vi "Teleop.vi"(0 "Call Context":T9) -> (13 "SubState 3":T1, 14 "SubState 0":T5=enum."driver control", 15 "Loop 1 Data":T6, 16 "Loop 0 Data":T7, 17 "SubState 1":T5, 18 "Loop 2 Data":T4, 19 "SubState 2":T5)   [LabVIEW 2014]
uses:
  typedefs/state machine/subStates.ctl
  <vilib>/Rock Robotics/WPI/DriverStation/WPI_DriverStationDerivedRobotMode.ctl
  typedefs/loop datatypes/Loop 0 Datatype.ctl
  typedefs/drive mode.ctl
  typedefs/loop datatypes/Loop 1 Datatype.ctl
  typedefs/loop datatypes/Loop 2 Datatype.ctl
  <vilib>/Rock Robotics/WPI/Joystick/WPI_JoystickDevRef.ctl
  <vilib>/Rock Robotics/WPI/Joystick/WPI_JoystickDeviceEnum.ctl
  typedefs/state machine/singleUseSubstate.ctl
  typedefs/fg_getset.ctl
  typedefs/vision/vision enable.ctl
  global variables/devrefs.vi
panel:
  out "Drive to DC":bool
  out "JS3":T2={"Device"=enum."USB 1"}
  out "JS1":T2={"Device"=enum."USB 1"}
  out "JS2":T2={"Device"=enum."USB 1"}
  out "Exit Value":i32=-1
  # "Teleoperated Loop Data and Substates"
  # "Drive Loop"
  # "Loop 1: Lift"
  # "Loop 2: Container Arm"
  # "Loop 3: Tote Pistons"
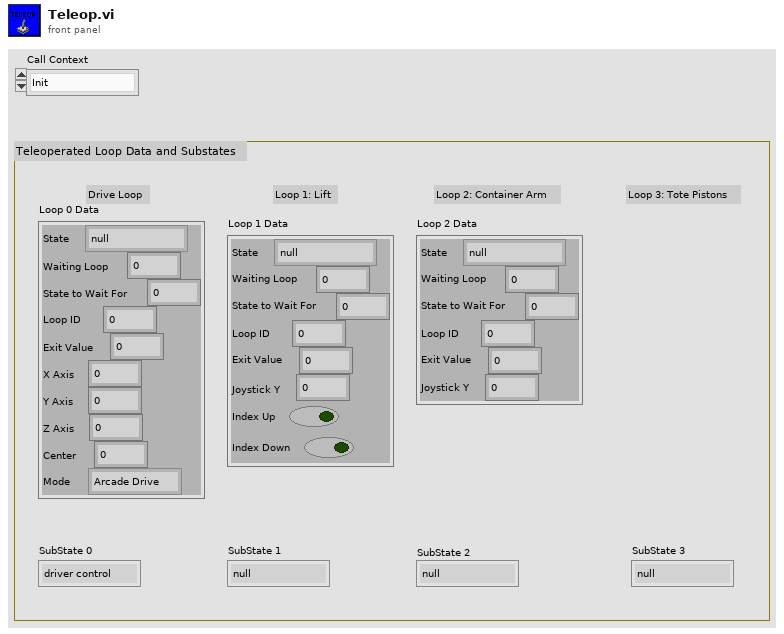
[diagram p1: front panel]
types:
  T1 = typedef "singleUseSubstate.ctl" = enum16{"null", "wait", "extend", "retract", "end"}
  T2 = typedef "WPI_JoystickDevRef.ctl" = cluster{"Device":T3}
  T3 = typedef "WPI_JoystickDeviceEnum.ctl" = enum16{"USB 0", "USB 1", "USB 2", "USB 3", "USB 4", "USB 5"}
  T4 = typedef "Loop 2 Datatype.ctl" = cluster{"State":T5, "Waiting Loop":i32, "State to Wait For":i32, "Loop ID":i32, "Exit Value":i32, "Joystick Y":dbl}
  T5 = typedef "subStates.ctl" = enum16{"null", "wait", "driver control", "auto", "manual override", "hold position", "rotate", "test", "end"}
  T6 = typedef "Loop 1 Datatype.ctl" = cluster{"State":T5, "Waiting Loop":i32, "State to Wait For":i32, "Loop ID":i32, "Exit Value":i32, "Joystick Y":dbl, "Index Up":bool, "Index Down":bool}
  T7 = typedef "Loop 0 Datatype.ctl" = cluster{"State":T5, "Waiting Loop":i32, "State to Wait For":i32, "Loop ID":i32, "Exit Value":i32, "X Axis":dbl, "Y Axis":dbl, "Z Axis":dbl, "Center":dbl, "Mode":T8}
  T8 = typedef "drive mode.ctl" = enum16{"Arcade Drive", "H-Drive", "H-Drive PID"}
  T9 = typedef "WPI_DriverStationDerivedRobotMode.ctl" = enum16{"Init", "Execute", "Stop"}
  T10 = cluster{"axis 1 (x)":dbl, "axis 2 (y)":dbl, "axis 3 (twist)":dbl, "axis 4 (throttle)":dbl, "axis 5":dbl, "axis 6":dbl}
  T11 = typedef "vision enable.ctl" = enum16{"Enable", "Disable", "Stop"}
  T12 = typedef "fg_getset.ctl" = enum16{"Get", "Set"}
  T13 = typedef "WPI_GyroDevRef.ctl" = cluster{"DevStatus":errorcluster, "Analog Module":T14, "Analog Channel":T15, "Offset":dbl, "Gain (VoltsPerDegree/Second)":dbl}
  T14 = typedef "FPGA_TypedefAnalogModule.ctl" = enum16{"Controller 1"}
  T15 = typedef "FPGA_AIChannel.ctl" = enum8{"AI 0", "AI 1", "AI 2", "AI 3", "AI MXP 0", "AI MXP 1", "AI MXP 2", "AI MXP 3", "Invalid"}
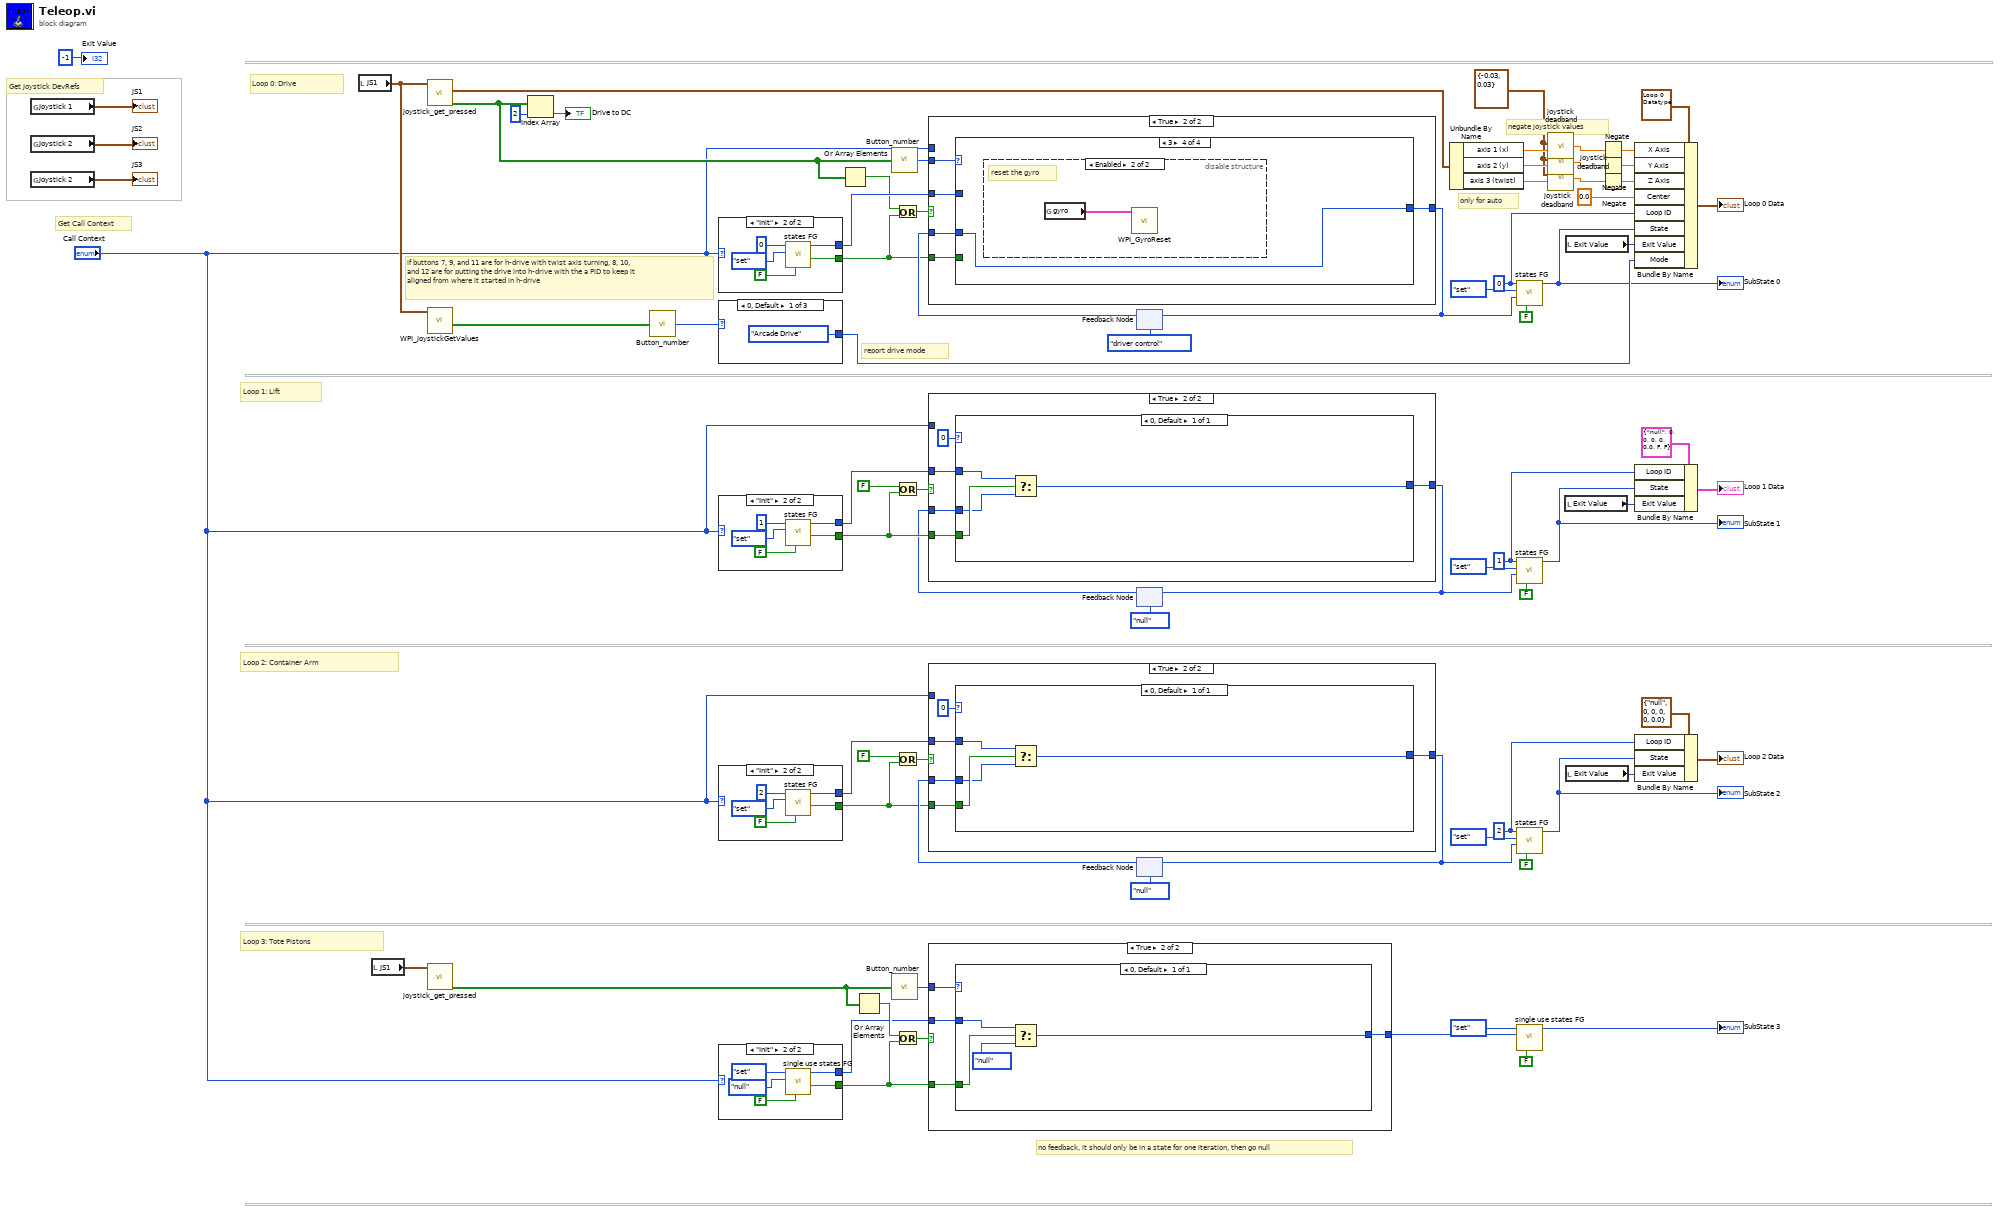
[diagram p0: block diagram]
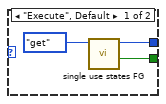
[diagram p2: hidden frame]
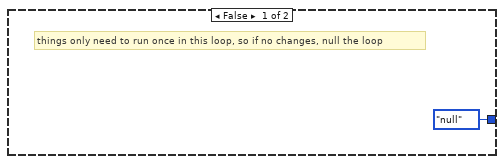
[diagram p3: hidden frame]
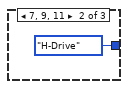
[diagram p4: hidden frame]
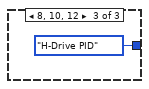
[diagram p5: hidden frame]
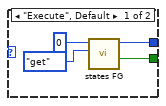
[diagram p6: hidden frame]
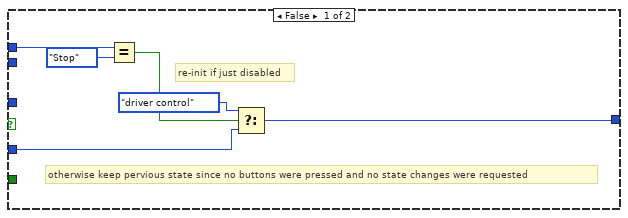
[diagram p7: hidden frame]
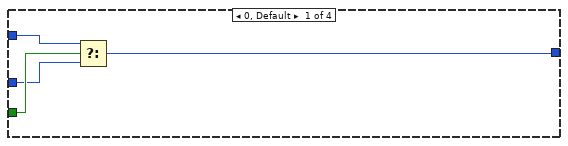
[diagram p8: hidden frame]
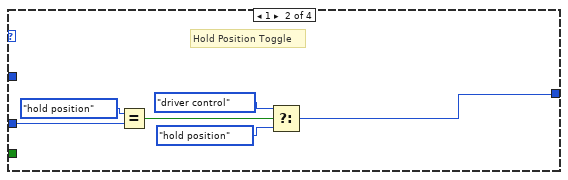
[diagram p9: hidden frame]
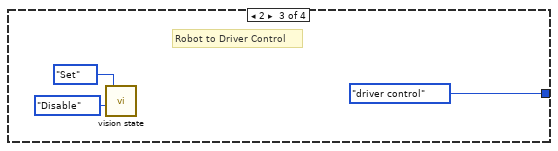
[diagram p10: hidden frame]
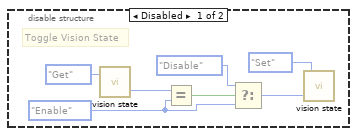
[diagram p11: hidden frame]
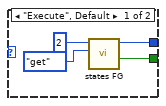
[diagram p12: hidden frame]
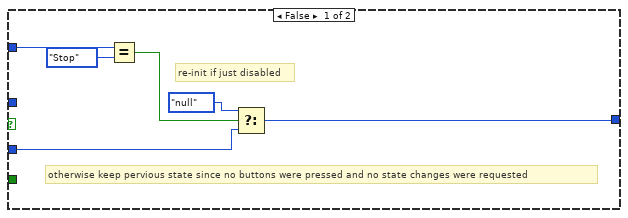
[diagram p13: hidden frame]
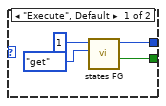
[diagram p14: hidden frame]
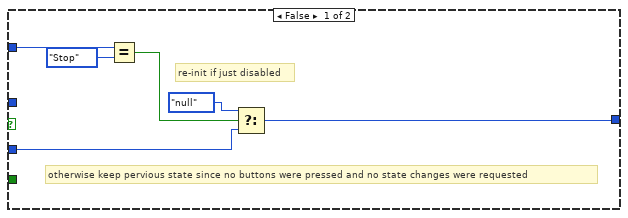
[diagram p15: hidden frame]
diagram:
  w2 = cluster{"Deadband Min":dbl, "Deadband Max":dbl} {"Deadband Min"=-0.03, "Deadband Max"=0.03} ("Deadband Range")
  w6 = 0 ("Loop ID")
  w61 = 2 ("Loop ID")
  w72 = 1 ("Loop ID")
  # "no feedback, it should only be in a state for one iteration, then go null"
  # "report drive mode"
  # "only for auto"
  # "if buttons 7, 9, and 11 are for h-drive with twist axis turning, 8, 10, \nand 12 are for putting the drive into h-drive with the a PID to keep it\naligned from where it started in h-drive"
  # "negate joystick values"
  # "Loop 3: Tote Pistons"
  # "Loop 2: Container Arm"
  # "Get Call Context"
  # "Get Joystick DevRefs"
  # "Loop 1: Lift"
  # "Loop 0: Drive"
  n1 = global read "devrefs.vi" "Joystick 1"() -> (→"JS1":T2)
  n2 = global read "devrefs.vi" "Joystick 2"() -> (→"JS2":T2)
  n3 = global read "devrefs.vi" "Joystick 2"() -> (→"JS3":T2)
  n4 = local read "JS1"() -> (w28:T2)
  n5 = local read "JS1"() -> (w22:T2)
  n6 = call "joystick_get_pressed.vi"("JoystickDevRef"=w28) -> ("Buttons Pressed?"=w29:bool[], "Axes"=w36:T10)  [unwired: 4 in, 3 out]
  n7 = call <vilib>:"WPI_JoystickGetValues.vi"("JoystickDevRef"=w28) -> ("Buttons"=w11:bool[])  [unwired: 6 in, 4 out]
  n8 = call "joystick_get_pressed.vi"("JoystickDevRef"=w22) -> ("Buttons Pressed?"=w21:bool[])  [unwired: 4 in, 4 out]
  n9 = Index Array(array=w29, index=2) -> (element=→"Drive to DC":bool)
  n10 = call "Button_number.vi"("Button Array"=w11) -> ("Button Pressed"=w10:i32)
  n11 = case shown="\"Init\"" "Call Context" {
    tunnel: [w80 w85] -> w47
    tunnel: [w79 w83] -> w51
    frame "Execute", Default {
      n12 = call "states FG.vi"("menu (get)"=enum16{"set", "get"}."get", "Loop ID"=0) -> ("exit out"=w80:bool, "subState out"=w79:T5)  [unwired: 6 in, 2 out]
    }
    frame "Init" {
      n13 = call "states FG.vi"("exit in"=FALSE, "menu (get)"=enum16{"set", "get"}."set", "Loop ID"=0) -> ("exit out"=w85:bool, "subState out"=w83:T5)  [unwired: 5 in, 2 out]
    }
  }
  n14 = case shown="0, Default" w10 {
    tunnel: [drive_mode."Arcade Drive" ("Mode") drive_mode."H-Drive" ("Mode") drive_mode."H-Drive PID" ("Mode")] -> w9
    frame 0, Default {
    }
    frame 7, 9, 11 {
    }
    frame 8, 10, 12 {
    }
  }
  n15 = case shown="\"Init\"" "Call Context" {
    tunnel: [w92 w97] -> w78
    tunnel: [w91 w95] -> w74
    frame "Execute", Default {
      n16 = call "states FG.vi"("menu (get)"=enum16{"set", "get"}."get", "Loop ID"=1) -> ("exit out"=w92:bool, "subState out"=w91:T5)  [unwired: 6 in, 2 out]
    }
    frame "Init" {
      n17 = call "states FG.vi"("exit in"=FALSE, "menu (get)"=enum16{"set", "get"}."set", "Loop ID"=1) -> ("exit out"=w97:bool, "subState out"=w95:T5)  [unwired: 5 in, 2 out]
    }
  }
  n18 = case shown="\"Init\"" "Call Context" {
    tunnel: [w101 w106] -> w56
    tunnel: [w100 w104] -> w60
    frame "Execute", Default {
      n19 = call "states FG.vi"("menu (get)"=enum16{"set", "get"}."get", "Loop ID"=2) -> ("exit out"=w101:bool, "subState out"=w100:T5)  [unwired: 6 in, 2 out]
    }
    frame "Init" {
      n20 = call "states FG.vi"("exit in"=FALSE, "menu (get)"=enum16{"set", "get"}."set", "Loop ID"=2) -> ("exit out"=w106:bool, "subState out"=w104:T5)  [unwired: 5 in, 2 out]
    }
  }
  n21 = case shown="\"Init\"" "Call Context" {
    tunnel: [w111 w115] -> w15
    tunnel: [w110 w116] -> w16
    frame "Execute", Default {
      n22 = call "single use states FG.vi"("menu (get)"=enum16{"set", "get"}."get") -> ("exit out"=w111:bool, "substate out"=w110:T1)  [unwired: 7 in, 2 out]
    }
    frame "Init" {
      n23 = call "single use states FG.vi"("exit in"=FALSE, "substate"=singleUseSubstate."null", "menu (get)"=enum16{"set", "get"}."set") -> ("exit out"=w115:bool, "substate out"=w116:T1)  [unwired: 5 in, 2 out]
    }
  }
  n24 = Or Array Elements(Boolean array=w29) -> (logical OR=w39:bool)
  n25 = Or Array Elements(Boolean array=w21) -> (logical OR=w18:bool)
  n26 = call "Button_number.vi"("Button Array"=w29) -> ("Button Pressed"=w40:i32)
  n27 = call "Button_number.vi"("Button Array"=w21) -> ("Button Pressed"=w19:i32)
  n28 = Or(x=w39, y=w47) -> (x .or. y?=w53:bool)
  n29 = Or(x=FALSE, y=w78) -> (x .or. y?=w67:bool)
  n30 = Or(x=FALSE, y=w56) -> (x .or. y?=w64:bool)
  n31 = Or(x=w18, y=w15) -> (x .or. y?=w17:bool)
  n32 = case shown="True" w17 {
    tunnel: [singleUseSubstate."null" ("substate out") w120] -> w20
    tunnel: w16 -> [_ w121]
    tunnel: w15 -> [_ w119]
    tunnel: w19 -> [_ w118]
    frame False {
      # "things only need to run once in this loop, so if no changes, null the loop"
    }
    frame True {
      n33 = case shown="0, Default" w118 {
        tunnel: w121 -> [w124]
        tunnel: [w123] -> w120
        tunnel: w119 -> [w125]
        frame 0, Default {
          n34 = Select(t=w124, s=w125, f=singleUseSubstate."null") -> (s? t:f=w123:T1)
        }
      }
    }
  }
  n35 = feedback #1(subStates."driver control" ("Drive SubState")) -> (w52:T5)
  n36 = case shown="True" w53 {
    tunnel: w52 -> [w128 w135]
    tunnel: [w126 w134] -> w35
    tunnel: w51 -> [_ w136]
    tunnel: w47 -> [_ w133]
    tunnel: "Call Context" -> [w131 _]
    tunnel: w40 -> [_ w132]
    frame False {
      # "re-init if just disabled"
      # "otherwise keep pervious state since no buttons were pressed and no state changes were requested"
      n37 = Equal?(x=w131, y=WPI_DriverStationDerivedRobotMode."Stop") -> (x = y?=w129:bool)
      n38 = Select(t=subStates."driver control", s=w129, f=w128) -> (s? t:f=w126:T5)
    }
    frame True {
      n39 = case shown="3" w132 {
        tunnel: w136 -> [w139 _ _ _]
        tunnel: w135 -> [w138 w146 _ w150]
        tunnel: [w137 w141 subStates."driver control" ("Drive SubState") w150] -> w134
        tunnel: w133 -> [w140 _ _ _]
        frame 0, Default {
          n40 = Select(t=w139, s=w140, f=w138) -> (s? t:f=w137:T5)
        }
        frame 1 {
          # "Hold Position Toggle"
          n41 = Equal?(x=subStates."hold position", y=w146) -> (x = y?=w144:bool)
          n42 = Select(t=subStates."driver control" ("Drive SubState"), s=w144, f=subStates."hold position" ("Drive SubState")) -> (s? t:f=w141:T5)
        }
        frame 2 {
          # "Robot to Driver Control"
          n43 = call "vision state.vi"("State In"=vision_enable."Disable" ("Action"), "Menu"=fg_getset."Set") -> ()  [unwired: 2 out]
        }
        frame 3 {
          n44 = disable-structure shown="Enabled" {
            frame Disabled {
              w155 = vision_enable."Enable" ("y")
              # "Toggle Vision State"
              n45 = call "vision state.vi"("Menu"=fg_getset."Get") -> ("State Out"=w153:T11)  [unwired: 1 in, 1 out]
              n46 = Equal?(x=w153, y=w155) -> (x = y?=w154:bool)
              n47 = Select(t=vision_enable."Disable" ("y"), s=w154, f=w155) -> (s? t:f=w157:T11)
              n48 = call "vision state.vi"("State In"=w157, "Menu"=fg_getset."Set") -> ()  [unwired: 2 out]
            }
            frame Enabled {
              # "reset the gyro"
              n49 = global read "devrefs.vi" "gyro"() -> (w158:T13)
              n50 = call <vilib>:"WPI_GyroReset.vi"("GyroDevRef"=w158) -> ()  [unwired: 9 in, 2 out]
            }
          }
        }
      }
    }
  }
  n51 = feedback-in #1(w35) -> ()
  n52 = feedback #2(subStates."null" ("Drive SubState")) -> (w68:T5)
  n53 = case shown="True" w67 {
    tunnel: w68 -> [w161 w168]
    tunnel: [w159 w167] -> w34
    tunnel: w74 -> [_ w169]
    tunnel: w78 -> [_ w166]
    tunnel: "Call Context" -> [w164 _]
    frame False {
      # "re-init if just disabled"
      # "otherwise keep pervious state since no buttons were pressed and no state changes were requested"
      n54 = Equal?(x=w164, y=WPI_DriverStationDerivedRobotMode."Stop") -> (x = y?=w162:bool)
      n55 = Select(t=subStates."null", s=w162, f=w161) -> (s? t:f=w159:T5)
    }
    frame True {
      n56 = case shown="0, Default" 0 ("Button Pressed") {
        tunnel: w169 -> [w172]
        tunnel: w168 -> [w171]
        tunnel: [w170] -> w167
        tunnel: w166 -> [w173]
        frame 0, Default {
          n57 = Select(t=w172, s=w173, f=w171) -> (s? t:f=w170:T5)
        }
      }
    }
  }
  n58 = feedback-in #2(w34) -> ()
  n59 = feedback #3(subStates."null" ("Drive SubState")) -> (w63:T5)
  n60 = case shown="True" w64 {
    tunnel: w63 -> [w176 w183]
    tunnel: [w174 w182] -> w33
    tunnel: w60 -> [_ w184]
    tunnel: w56 -> [_ w181]
    tunnel: "Call Context" -> [w179 _]
    frame False {
      # "re-init if just disabled"
      # "otherwise keep pervious state since no buttons were pressed and no state changes were requested"
      n61 = Equal?(x=w179, y=WPI_DriverStationDerivedRobotMode."Stop") -> (x = y?=w177:bool)
      n62 = Select(t=subStates."null", s=w177, f=w176) -> (s? t:f=w174:T5)
    }
    frame True {
      n63 = case shown="0, Default" 0 ("Button Pressed") {
        tunnel: w184 -> [w187]
        tunnel: w183 -> [w186]
        tunnel: [w185] -> w182
        tunnel: w181 -> [w188]
        frame 0, Default {
          n64 = Select(t=w187, s=w188, f=w186) -> (s? t:f=w185:T5)
        }
      }
    }
  }
  n65 = feedback-in #3(w33) -> ()
  n66 = Unbundle By Name(w36) -> ("axis 1 (x)"=w27:dbl, "axis 2 (y)"=w26:dbl, "axis 3 (twist)"=w1:dbl)
  n67 = call "states FG.vi"("exit in"=FALSE, "subState in"=w35, "menu (get)"=enum16{"set", "get"}."set", "Loop ID"=w6) -> ("subState out"=w7:T5)  [unwired: 4 in, 3 out]
  "SubState 0" <- w7
  n68 = call "states FG.vi"("exit in"=FALSE, "subState in"=w34, "menu (get)"=enum16{"set", "get"}."set", "Loop ID"=w72) -> ("subState out"=w37:T5)  [unwired: 4 in, 3 out]
  "SubState 1" <- w37
  n69 = call "states FG.vi"("exit in"=FALSE, "subState in"=w33, "menu (get)"=enum16{"set", "get"}."set", "Loop ID"=w61) -> ("subState out"=w38:T5)  [unwired: 4 in, 3 out]
  "SubState 2" <- w38
  n70 = call "single use states FG.vi"("exit in"=FALSE, "substate"=w20, "menu (get)"=enum16{"set", "get"}."set") -> ("substate out"=→"SubState 3":T1)  [unwired: 5 in, 3 out]
  n71 = call "joystick deadband.vi"("Joystick In"=w27, "Deadband Range"=w2) -> ("Joystick Out"=w24:dbl)  [unwired: 4 in]
  n72 = call "joystick deadband.vi"("Joystick In"=w26, "Deadband Range"=w2) -> ("Joystick Out"=w25:dbl)  [unwired: 4 in]
  n73 = call "joystick deadband.vi"("Joystick In"=w1, "Deadband Range"=w2) -> ("Joystick Out"=w4:dbl)  [unwired: 4 in]
  n74 = local read "Exit Value"() -> (w70:i32)
  n75 = local read "Exit Value"() -> (w8:i32)
  n76 = local read "Exit Value"() -> (w62:i32)
  n77 = Negate(x=w24) -> (-x=w42:dbl)
  n78 = Negate(x=w25) -> (-x=w41:dbl)
  n79 = Negate(x=w4) -> (-x=w3:dbl)
  n80 = Bundle By Name(cluster=T7 {"State"=enum."null", "Waiting Loop"=0, "State to Wait For"=0, "Loop ID"=0, "Exit Value"=0, "X Axis"=0.0, "Y Axis"=0.0, "Z Axis"=0.0, "Center"=0.0, "Mode"=enum."Arcade Drive"} ("Cluster"), "X Axis"=w42, "Y Axis"=w41, "Z Axis"=w3, "Center"=0.0, "Loop ID"=w6, "State"=w7, "Exit Value"=w8, "Mode"=w9) -> (→"Loop 0 Data":T7)
  n81 = Bundle By Name(cluster=T6 {"State"=enum."null", "Waiting Loop"=0, "State to Wait For"=0, "Loop ID"=0, "Exit Value"=0, "Joystick Y"=0.0, "Index Up"=FALSE, "Index Down"=FALSE} ("Cluster"), "Loop ID"=w72, "State"=w37, "Exit Value"=w70) -> (→"Loop 1 Data":T6)
  n82 = Bundle By Name(cluster=T4 {"State"=enum."null", "Waiting Loop"=0, "State to Wait For"=0, "Loop ID"=0, "Exit Value"=0, "Joystick Y"=0.0} ("Loop 2 Data"), "Loop ID"=w61, "State"=w38, "Exit Value"=w62) -> (→"Loop 2 Data":T4)
  "Exit Value" <- -1 ("Exit Value")
